vi "Make amp sweep signal.vi"(0 "nsamp":dbl, 1 "stimdur":dbl, 2 "Output freq (Hz)":dbl, 3 "sinfreq":dbl, 4 "sinamp start":dbl, 5 "sinamp end":dbl, 6 "noiseamp start":dbl, 7 "beforedur":dbl, 8 "noiseamp end":dbl, 9 "afterdur":dbl, 10 "hicutoff":dbl, 12 "lowcutoff":dbl) -> (14 "Stimulus out":T2={"type"=enum."Zero", "sinfreq start"=0.0, "sinfreq end"=0.0, "sinamp start"=0.0, "sinamp end"=0.0, "noise freq lo"=0.0, "noise freq hi"=0.0, "noiseamp start"=0.0, "noiseamp end"=0.0, "stimdur"=0.0, "before dur"=0.0, "after dur"=0.0, "pulse data"={"time"=[], "phase/vel"=[], "dir/shift"=[], "amplitude"=[], "duration"=[]}} {"noise freq hi" min=0.0 step=0.5; "noise freq lo" min=0.0 step=0.5; "noiseamp end" min=0.0 step=0.5; "noiseamp start" min=0.0 step=0.5}, 15 "sine wave":dbl[](array[numeric]), 16 "noise":dbl[](array[numeric]), 17 "phases":T1)   [LabVIEW 2013]
uses:
  Stimulus.ctl
  Stimulus type.ctl
  Pulse data.ctl
  Phases.ctl
  <vilib>/Analysis/1siggen.llb/Ramp Pattern by Samples.vi
  <vilib>/Analysis/NI_AALBase.lvlib
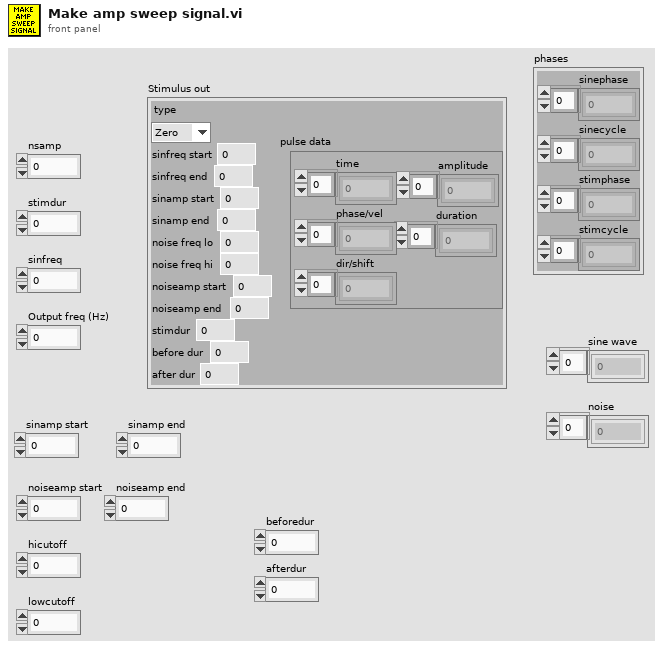
[diagram p1: front panel]
types:
  T1 = typedef "Phases.ctl" = cluster{"sinephase":dbl[], "sinecycle":dbl[], "stimphase":dbl[], "stimcycle":dbl[]}
  T2 = typedef "Stimulus.ctl" = cluster{"type":T3, "sinfreq start":dbl, "sinfreq end":dbl, "sinamp start":dbl, "sinamp end":dbl, "noise freq lo":dbl, "noise freq hi":dbl, "noiseamp start":dbl, "noiseamp end":dbl, "stimdur":dbl, "before dur":dbl, "after dur":dbl, "pulse data":T4}
  T3 = typedef "Stimulus type.ctl" = enum16{"Sine", "Zero", "Frequency sweep", "Two frequency", "Amplitude sweep", "Pulses", "Shifts", "Ramps"}
  T4 = typedef "Pulse data.ctl" = cluster{"time":dbl[], "phase/vel":dbl[], "dir/shift":dbl[], "amplitude":dbl[], "duration":dbl[]}
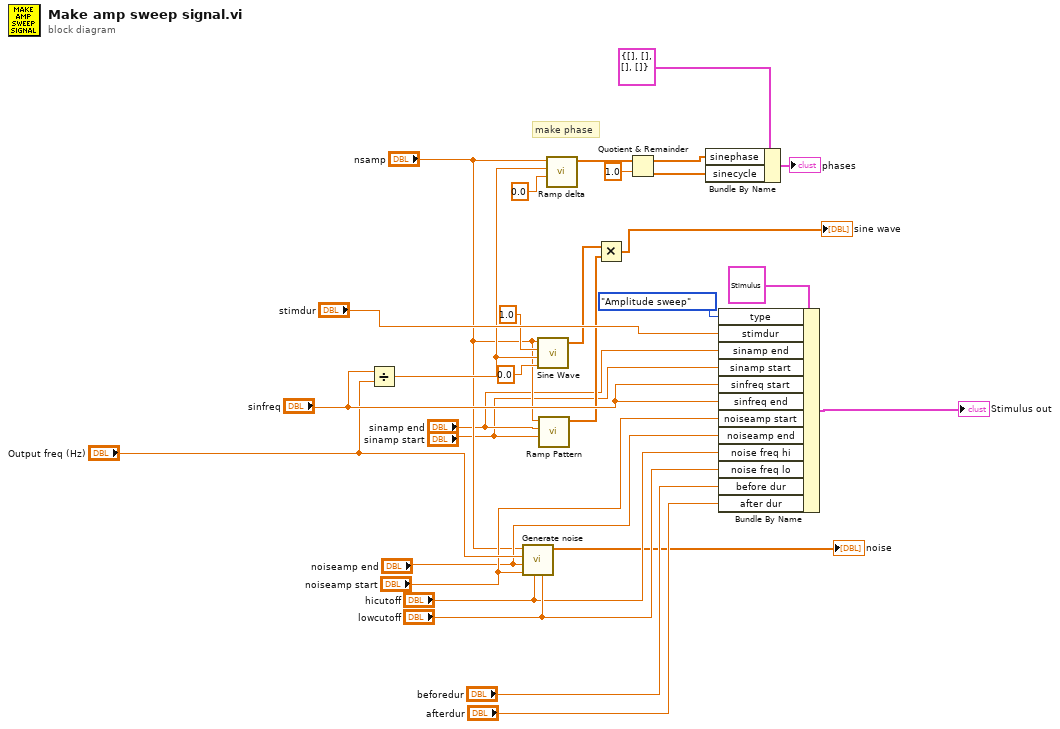
[diagram p0: block diagram]
diagram:
  # "make phase"
  n1 = Divide(x="sinfreq", y="Output freq (Hz)") -> (x/y=w17:dbl)
  n2 = call "Generate noise.vi"("lo cutoff"="lowcutoff", "hi cutoff"="hicutoff", "start amplitude"="noiseamp start", "end amplitude"="noiseamp end", "sampling freq"="Output freq (Hz)", "samples"="nsamp") -> ("noise"=→"noise":dbl[])  [unwired: 5 in]
  n3 = call <vilib>:"Sine Wave.vi"("samples"="nsamp", "amplitude"=1.0, "frequency"=w17, "phase in"=0.0) -> ("sine wave"=w5:dbl[])  [unwired: 1 in, 2 out]
  n4 = call-poly <vilib>:"Ramp Pattern.vi"("start"="sinamp start", "end"="sinamp end", "samples"="nsamp") -> ("Ramp Pattern"=w4:dbl[])  [unwired: 7 in, 1 out]
  n5 = call "Ramp delta.vi"("start"=0.0, "delta"=w17, "samples"="nsamp") -> ("ramp signal"=w15:dbl[])  [unwired: 7 in, 1 out]
  n6 = Multiply(x=w5, y=w4) -> (x*y=→"sine wave":dbl[])
  n7 = Quotient & Remainder(x=w15, y=1.0 ("start")) -> (x-y*floor(x/y)=w12:dbl[], floor(x/y)=w11:dbl[])
  n8 = Bundle By Name(cluster=T1 {"sinephase"=[], "sinecycle"=[], "stimphase"=[], "stimcycle"=[]} ("phases"), "sinephase"=w12, "sinecycle"=w11) -> (→"phases":T1)
  n9 = Bundle By Name(cluster=T2 {"type"=enum."Zero", "sinfreq start"=0.0, "sinfreq end"=0.0, "sinamp start"=0.0, "sinamp end"=0.0, "noise freq lo"=0.0, "noise freq hi"=0.0, "noiseamp start"=0.0, "noiseamp end"=0.0, "stimdur"=0.0, "before dur"=0.0, "after dur"=0.0, "pulse data"={"time"=[], "phase/vel"=[], "dir/shift"=[], "amplitude"=[], "duration"=[]}} ("Stimulus 2"), "type"=Stimulus_type."Amplitude sweep", "stimdur"="stimdur", "sinamp end"="sinamp end", "sinamp start"="sinamp start", "sinfreq start"="sinfreq", "sinfreq end"="sinfreq", "noiseamp start"="noiseamp start", "noiseamp end"="noiseamp end", "noise freq hi"="hicutoff", "noise freq lo"="lowcutoff", "before dur"="beforedur", "after dur"="afterdur") -> (→"Stimulus out":T2)
